vi "Initialize HLA helpers.vi"(8 "error in":errorcluster) -> (0 "error out":errorcluster, 3 "hla map helpers":T1)   [LabVIEW 2019, in "HLA Custom Device Engine.lvlib"]
uses:
  HLA Custom Device Engine.lvlib
  RThlaMapHelpers.ctl
  map_object.ctl
  map_attribute.ctl
  map_attribute_data.ctl
  emea-ni-adg-hla-lv/src/library/typedefs/hla_vendor_type.ctl
  emea-ni-adg-hla-lv/src/helpers/Attribute Handle Value Map/ahvm.lvlib
  emea-ni-adg-hla-lv/src/helpers/Parameter Handle Value Map/phvm.lvlib
  emea-ni-adg-hla-lv/src/helpers/Attribute Handle Set/ahs.lvlib
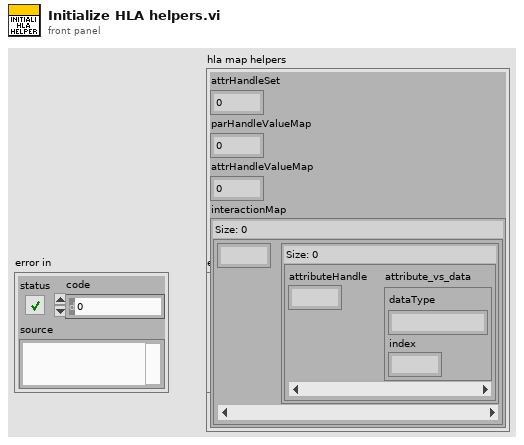
[diagram p1: front panel]
types:
  T1 = typedef "RThlaMapHelpers.ctl" = cluster{"attrHandleSet":u64, "parHandleValueMap":u64, "attrHandleValueMap":u64, "interactionMap":T2}
  T2 = typedef "HLA Custom Device Engine.lvlib/map_object.ctl" = map{u64, T3}
  T3 = typedef "HLA Custom Device Engine.lvlib/map_attribute.ctl" = map{u64, T4}
  T4 = typedef "HLA Custom Device Engine.lvlib/map_attribute_data.ctl" = cluster{"dataType":string, "index":i32}
  T5 = typedef "hla_vendor_type.ctl" = enum16{"OpenRTI", "MAK"}
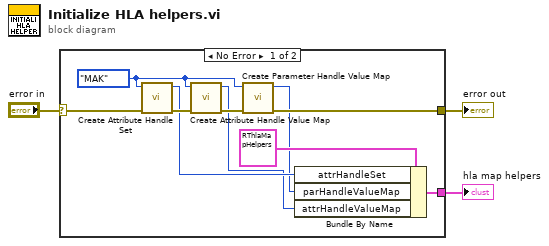
[diagram p0: block diagram]
diagram:
  n1 = case shown="No Error" "error in" {
    selector: "error in" -> [w9 w14]
    tunnel: [w10 w14] -> w3
    tunnel: [w7 _] -> w1
    frame No Error {
      w13 = hla_vendor_type."MAK" ("vendor")
      n2 = call "Create Attribute Handle Set.vi"("error in"=w9, "vendor"=w13) -> ("error out"=w11:errorcluster, "attrHandleSet"=w6:u64)  [unwired: 8 in]
      n3 = call "Create Attribute Handle Value Map.vi"("error in"=w11, "vendor"=w13) -> ("error out"=w12:errorcluster, "attrHandleValueMap"=w4:u64)  [unwired: 8 in]
      n4 = call "Create Parameter Handle Value Map.vi"("error in"=w12, "vendor"=w13) -> ("error out"=w10:errorcluster, "parHandleValueMap"=w5:u64)  [unwired: 8 in]
      n5 = Bundle By Name(cluster=T1 {"attrHandleSet"=0, "parHandleValueMap"=0, "attrHandleValueMap"=0, "interactionMap"={}}, "attrHandleSet"=w6, "parHandleValueMap"=w5, "attrHandleValueMap"=w4) -> (w7:T1)
    }
    frame Error {
    }
  }
  "error out" <- w3
  "hla map helpers" <- w1
